vi "Configure Analyzer.vi"(6 "Center Frequency (900MHz)":dbl=900000000.0 format="%#.9p", 7 "Margin (0.0)":dbl format="%^.3e", 8 "error in (no error)":errorcluster, 9 "Expected Nominal Power (0.0)":dbl format="%^.3e", 10 "Instance (1)":i32=1 format="%.0g", 11 "VISA resource name":refnum<visa-resource-name>) -> (0 "error out":errorcluster, 3 "VISA resource name out":refnum<visa-resource-name>)   [LabVIEW 2020, in "Rohde&Schwarz CMXP GPRF.lvlib"]
doc: "Configures the RF input path.\n\nAttributes:\nRSCMXPGPRF_ATTR_ANALYZER_EXPECTED_NOMINAL_POWER\nRSCMXPGPRF_ATTR_ANALYZER_USER_MARGIN\nRSCMXPGPRF_ATTR_ANALYZER_CENTER_FREQUENCY\n\nRemote-control commands:\nCONFigure:GPRF:MEAS<i>:RFSettings:ENPower\nCONFigure:GPRF:MEAS<i>:RFSettings:UMARgin\nCONFigure:GPRF:MEAS<i>:RFSettings:FREQuency"
uses:
  <instrlib>/Rohde&Schwarz CMXP GPRF/Rohde&Schwarz CMXP GPRF.lvlib
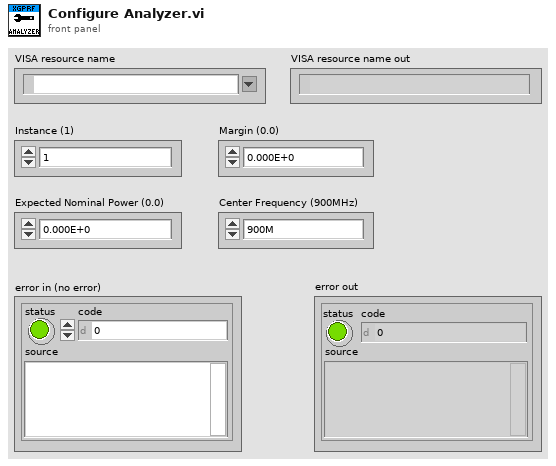
[diagram p1: front panel]
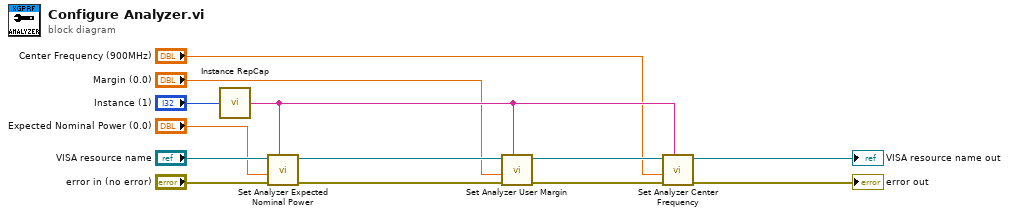
[diagram p0: block diagram]
diagram:
  n1 = call <instrlib>:"Instance RepCap.vi"("Instance in"="Instance (1)") -> ("Instance out"=w4:string)
  n2 = call "Set Analyzer Expected Nominal Power"("Repeated Capabilities"=w4, "error in (no error)"="error in (no error)", "Analyzer Expected Nominal Power (0.0)"="Expected Nominal Power (0.0)", "instrument handle"="VISA resource name") -> ("error out"=w10:errorcluster, "instrument handle out"=w9:refnum<visa-resource-name>)  [unwired: 6 in]
  n3 = call "Set Analyzer User Margin"("Repeated Capabilities"=w4, "error in (no error)"=w10, "Analyzer User Margin (0.0)"="Margin (0.0)", "instrument handle"=w9) -> ("error out"=w8:errorcluster, "instrument handle out"=w7:refnum<visa-resource-name>)  [unwired: 6 in]
  n4 = call "Set Analyzer Center Frequency"("Repeated Capabilities"=w4, "error in (no error)"=w8, "Analyzer Center Frequency (0.0)"="Center Frequency (900MHz)", "instrument handle"=w7) -> ("error out"=→"error out":errorcluster, "instrument handle out"=→"VISA resource name out":refnum<visa-resource-name>)  [unwired: 6 in]
